vi "Average_Temp.vi"() -> ()   [LabVIEW 2019]
panel:
  in  "stop":bool
  out "Thermometer":dbl(slide) scale=0.0..100.0
  out "Average Temp":dbl
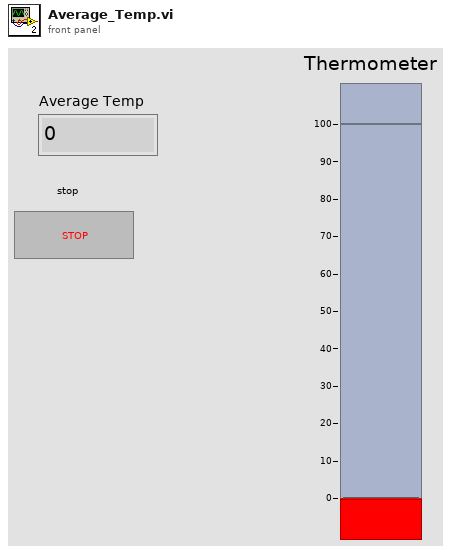
[diagram p1: front panel]
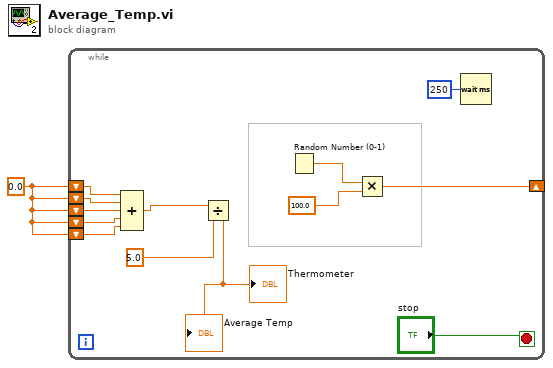
[diagram p0: block diagram]
diagram:
  w1 = 0.0
  n1 = while {
    shift-right: [w12] -> _
    shift-left: w1 -> [w7]
    shift-left: w1 -> [w6]
    shift-left: w1 -> [w5]
    shift-left: w1 -> [w4]
    shift-left: w1 -> [w3]
    stop <- "stop" stop-if-true
    n2 = Compound Arithmetic op=ADD(w7, w6, w5, w4, w3) -> (w2:dbl)
    n3 = Divide(x=w2, y=5.0) -> (x/y=→"Average Temp" →"Thermometer":dbl)
    n4 = Random Number (0-1)() -> (number: 0 to 1=w14:dbl)
    n5 = Multiply(x=w14, y=100.0) -> (x*y=w12:dbl)
    n6 = Wait (ms)(milliseconds to wait=u32 250) -> ()  [unwired: 1 out]
  }
